vi "Add LS State.vi"(8 "error in":errorcluster, 11 "PIOD in":refnum<class "PIOD.lvclass">) -> (0 "error out":errorcluster, 3 "PIOD out":refnum<class "PIOD.lvclass">)   [LabVIEW 2018, in "PIOD.lvlib" / "PIOD.lvclass"]
uses:
  PIOD.lvclass
  PPLs/PLC/Parent/PLC.lvlibp/PLC.lvclass
  PPLs/PLC/Light Stack/Light Stack.lvlibp/Light Stack.lvclass
  C:/AME Test Engineering/LabVIEW/PPLs/PLC/Parent/PLC.lvlibp/PLC.lvclass
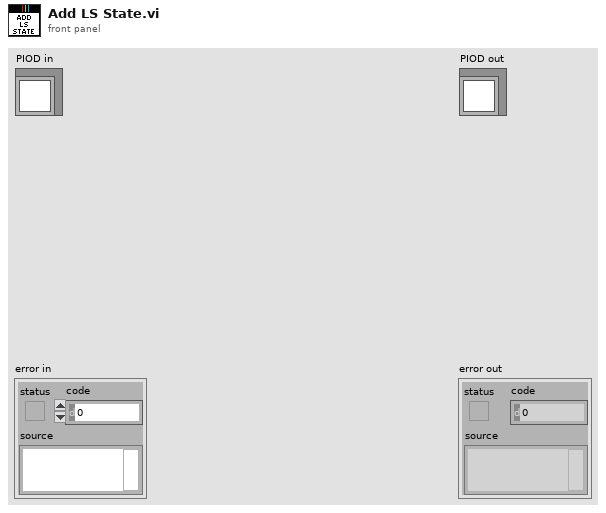
[diagram p1: front panel]
types:
  T1 = typedef "Light Stack.lvlibp/Light Mode.ctl" = enum16{"OFF", "ON", "BLINK"}
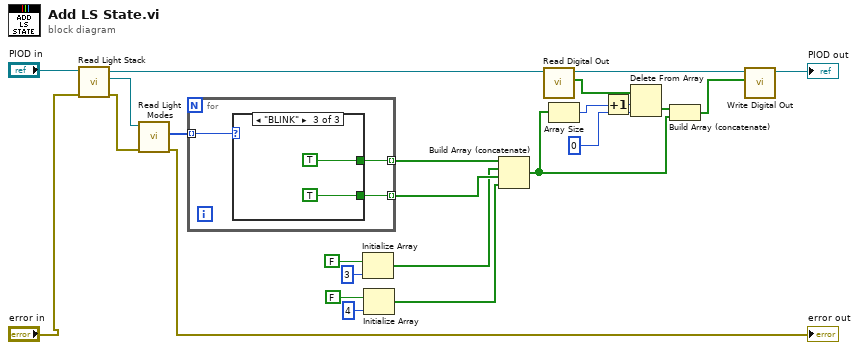
[diagram p0: block diagram]
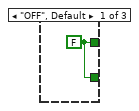
[diagram p2: hidden frame]
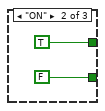
[diagram p3: hidden frame]
diagram:
  n1 = call "Read Light Stack.vi"("error in (no error)"="error in", "PLC in"="PIOD in") -> ("error out"=w22:errorcluster, "Light Stack"=w23:refnum<class "Light Stack.lvclass">, "PLC out"=w14:refnum<class "PIOD.lvclass">)  [unwired: 7 in]
  n2 = call "Read Light Modes.vi"("error in (no error)"=w22, "Light Stack in"=w23) -> ("error out"=→"error out":errorcluster, "Light Modes"=w20:T1[])  [unwired: 7 in, 1 out]
  n3 = for {
    tunnel: w20 -> [w27] mode=indexing
    tunnel: [w26] -> w15 mode=indexing
    tunnel: [w25] -> w16 mode=indexing
    n4 = case shown="\"BLINK\"" w27 {
      tunnel: [w28 FALSE TRUE] -> w26
      tunnel: [w28 TRUE TRUE] -> w25
      frame "OFF", Default {
        w28 = FALSE
      }
      frame "ON" {
      }
      frame "BLINK" {
      }
    }
  }
  n5 = Initialize Array(FALSE, 3 ("dimension size")) -> (w3:bool[])
  n6 = Initialize Array(FALSE, 4 ("dimension size")) -> (w2:bool[])
  n7 = Build Array (concatenate)(w16, w3, w15, w2) -> (w9:bool[])
  n8 = call "Read Digital Out.vi"("PLC in"=w14) -> ("Digital Out"=w13:bool[], "PLC out"=w10:refnum<class "PIOD.lvclass">)  [unwired: 8 in, 1 out]
  n9 = Array Size(array=w9) -> (size(s)=w6:i32)
  n10 = Increment(x=w6) -> (x+1=w1:i32)
  n11 = Delete From Array(array=w13, length=w1, index=0) -> (deleted portion=w8:bool[])  [unwired: 1 out]
  n12 = Build Array (concatenate)(w8, w9) -> (w12:bool[])
  n13 = call "Write Digital Out.vi"("Digital Out"=w12, "PLC in"=w10) -> ("PLC out"=→"PIOD out":refnum<class "PIOD.lvclass">)  [unwired: 8 in, 1 out]
